vi "test Estimate All Positions Swarm Method.vi"(8 "error in (no error)":errorcluster, 11 "TestCase in":refnum<class "Position Estimation Tests.lvclass">) -> (0 "error out":errorcluster, 3 "TestCase out":refnum<class "Position Estimation Tests.lvclass">)   [LabVIEW 2014, in "Position Estimation Tests.lvclass"]
uses:
  Position Estimation Tests.lvclass
  <vilib>/addons/_JKI Toolkits/VI Tester/TestCase.llb/TestCase.lvclass
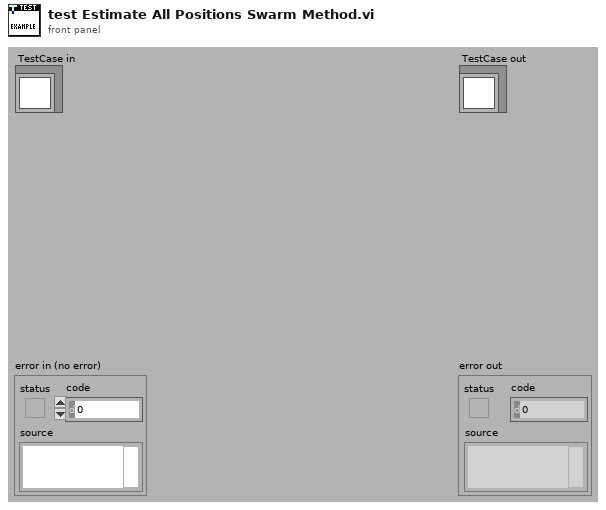
[diagram p1: front panel]
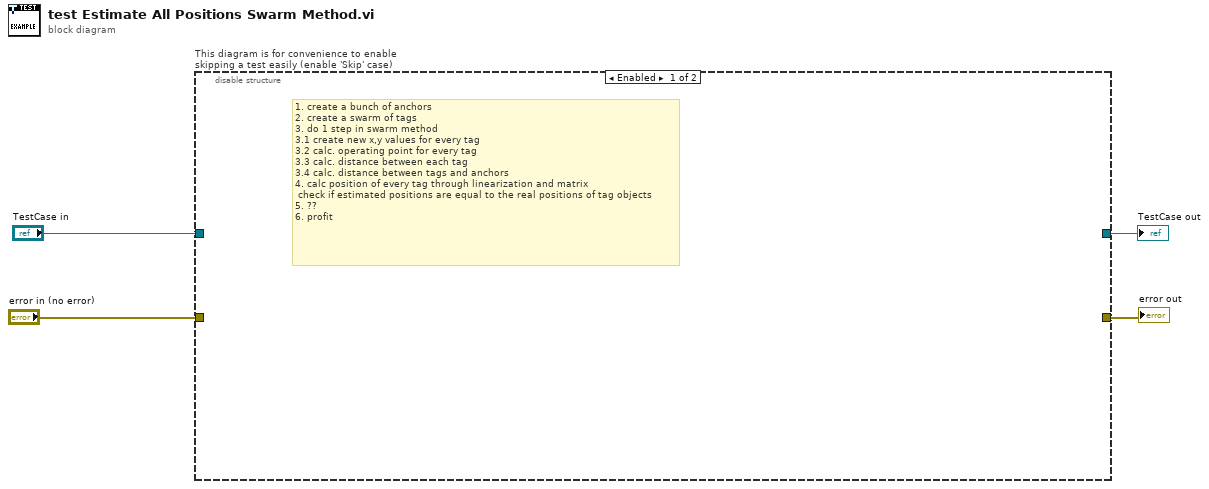
[diagram p0: block diagram]
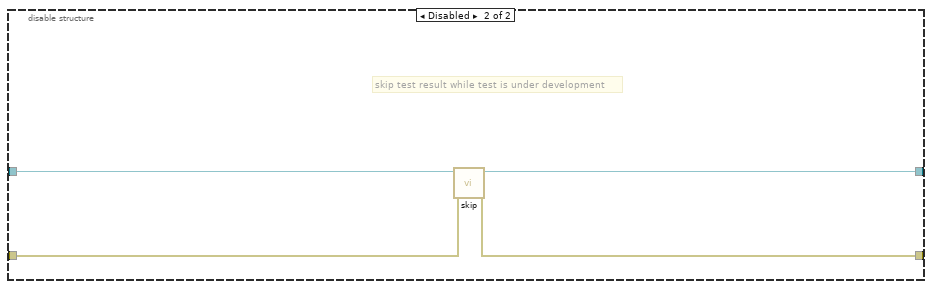
[diagram p2: hidden frame]
diagram:
  n1 = disable-structure "This diagram is for convenience to enable skipping a test easily (enable 'Skip' case)" shown="Enabled" {
    disable-tunnel: "TestCase in" -> [_ w8]
    disable-tunnel: [_ w6] -> w1
    disable-tunnel: [_ w7] -> w3
    disable-tunnel: "error in (no error)" -> [_ w5]
    frame Enabled {
      # "1. create a bunch of anchors\n2. create a swarm of tags\n3. do 1 step in swarm method\n3.1 create new x,y values for every tag\n3.2 calc. operating point for every tag\n3.3 calc. distance between each tag\n3.4 calc. distance between tags and anchors\n4. calc position of every tag through linearization and matrix\n check if estimated positions are equal to the real positions of tag objects\n5. ??\n6. profit"
    }
    frame Disabled {
      # "skip test result while test is under development"
      n2 = call <vilib>:"skip.vi"("error in (no error)"=w5, "TestCase in"=w8) -> ("error out"=w7:errorcluster, "TestCase out"=w6:refnum<class "Position Estimation Tests.lvclass">)  [unwired: 8 in]
    }
  }
  "error out" <- w3
  "TestCase out" <- w1
